vi "CalcShifts.vi"(0 "Sampling Rate (Hz)":dbl=1000000000.0, 1 "c (m/s)":i16=1485, 2 "delay (mm)":sgl, 3 "rf pts":i32, 5 "ROC (m)":dbl=0.012, 7 "# Elements":i16=5, 9 "Radii (m)":sgl[](array[numeric])=[0.0, 0.00132, 0.00142, 0.0019, 0.002, 0.00236, 0.00245, 0.00275, 0.00285, 0.0031], 11 "One Way Receive":bool, 12 "Focal lengths (m)":dbl[](array[numeric])=[0.0085, 0.009, 0.0095, 0.01, 0.0105, 0.011, 0.0115, 0.012, 0.0125, 0.013, 0.0135, 0.014, 0.0145, 0.015], 13 "File index number":i32, 14 "Dual mode":bool) -> (6 "ZoneStart":sgl[](array[numeric]), 8 "ZoneShift":sgl[](array[numeric]), 10 "ZoneLength":sgl[](array[numeric]), 15 "IndexVals":sgl[](array[numeric]))   [LabVIEW 2022 SP3]
panel:
  out "output variable":dbl
  in  "shift":i32
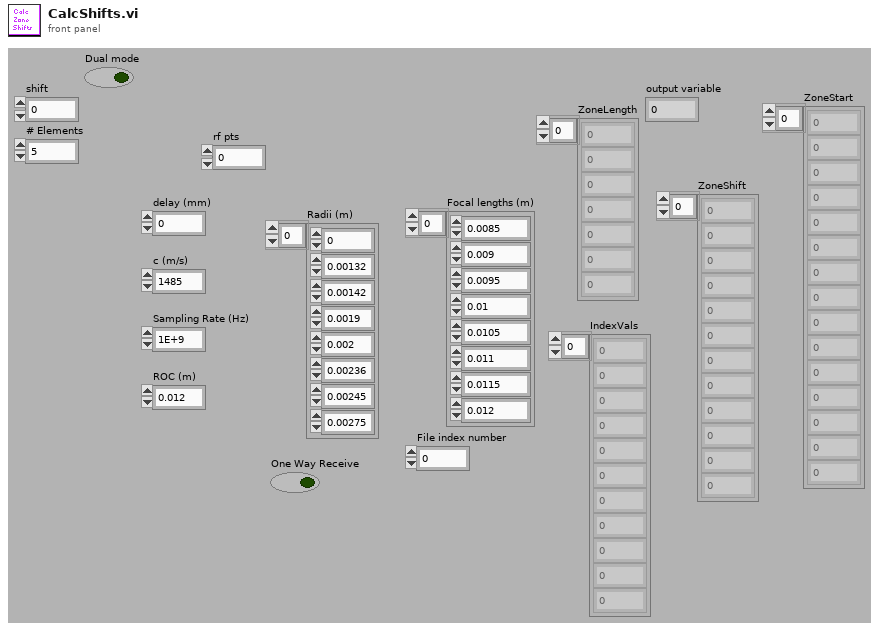
[diagram p1: front panel]
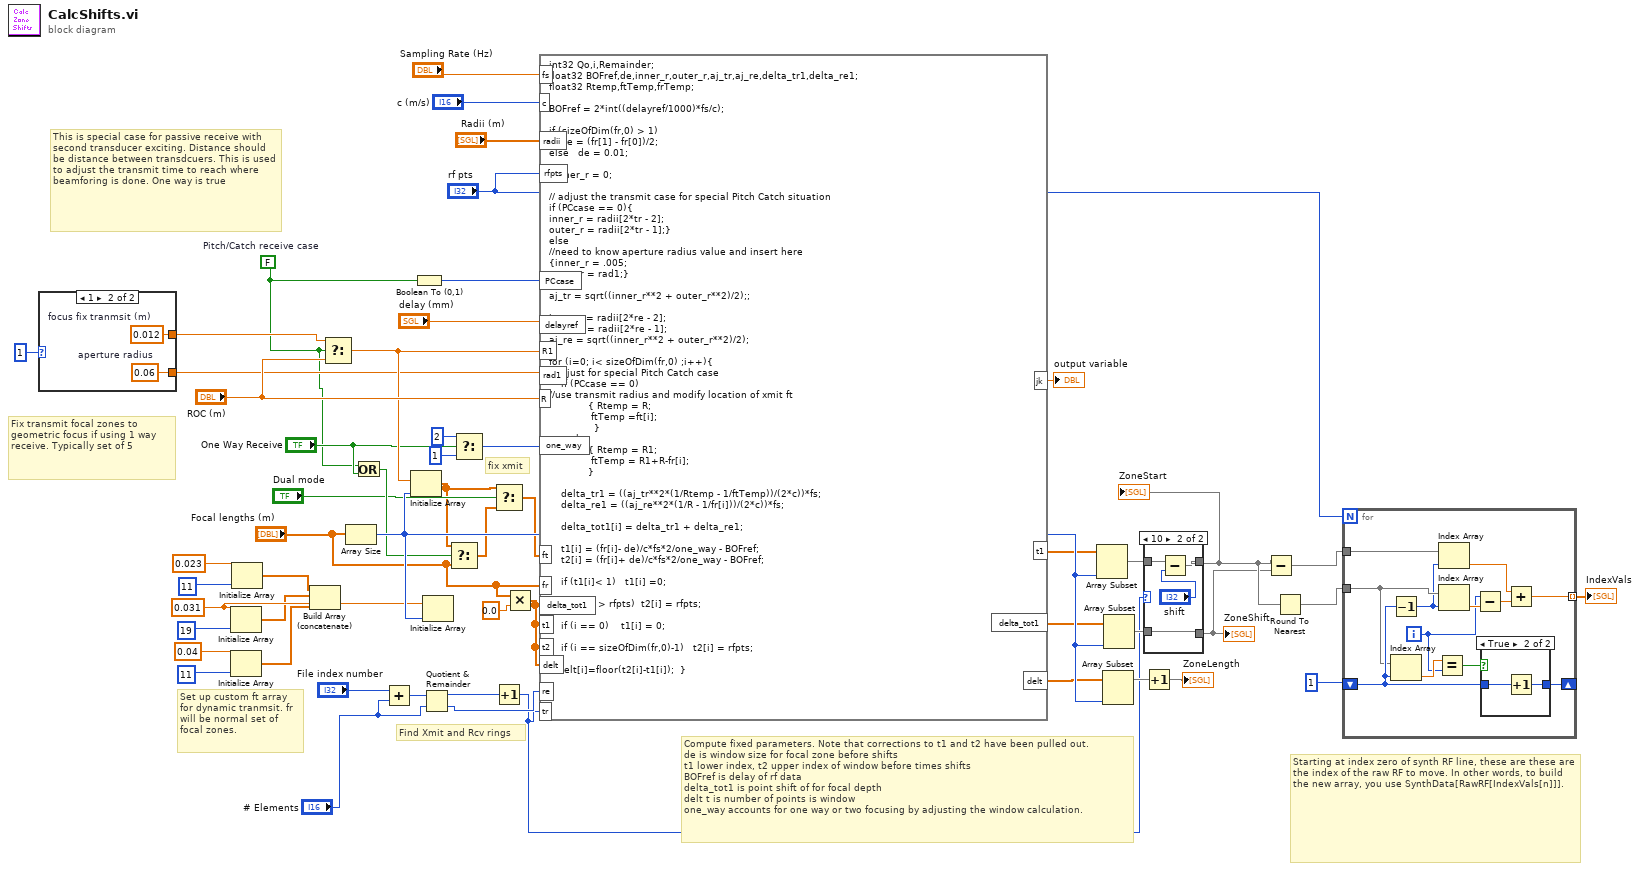
[diagram p0: block diagram]
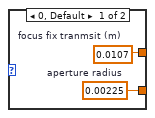
[diagram p2: hidden frame]
diagram:
  w7 = FALSE  # Pitch/Catch receive case
  w50 = 0.031
  # "fix xmit"
  # "This is special case for passive receive with second transducer exciting. Distance should be distance between transdcuers. This is used to adjust the transmit time to reach where beamforing is done. One way is true"
  # "Starting at index zero of synth RF line, these are these are the index of the raw RF to move. In other words, to build the new array, you use SynthData[RawRF[IndexVals[n]]]."
  # "Fix transmit focal zones to geometric focus if using 1 way receive. Typically set of 5"
  # "Set up custom ft array for dynamic tranmsit. fr will be normal set of focal zones."
  # "Find Xmit and Rcv rings"
  # "Compute fixed parameters. Note that corrections to t1 and t2 have been pulled out.\nde is window size for focal zone before shifts\nt1 lower index, t2 upper index of window before times shifts\nBOFref is delay of rf data\ndelta_tot1 is point shift of for focal depth\ndelt t is number of points is window\none_way accounts for one way or two focusing by adjusting the window calculation."
  n1 = case shown="1" 1 {
    tunnel: [w56 w58] -> w14
    tunnel: [w55 w57] -> w12
    frame 0, Default {
      w55 = 0.00225  # aperture radius
      w56 = 0.0107  # focus fix tranmsit (m)
    }
    frame 1 {
      w57 = 0.06  # aperture radius
      w58 = 0.012  # focus fix tranmsit (m)
    }
  }
  n2 = Initialize Array(w50, 19) -> (w48:dbl[])
  n3 = Initialize Array(0.04, 11) -> (w49:dbl[])
  n4 = Initialize Array(0.023, 11) -> (w47:dbl[])
  n5 = Build Array (concatenate)(w47, w48, w49) -> ()  [unwired: 1 out]
  n6 = Select(t=w14, s=w7, f="ROC (m)") -> (s? t:f=w16:dbl)
  n7 = Array Size(array="Focal lengths (m)") -> (size(s)=w52:i32)
  n8 = Or(x=w7, y="One Way Receive") -> (x .or. y?=w9:bool)
  n9 = Add(x="File index number", y="# Elements") -> (x+y=w39:i32)
  n10 = Initialize Array(w16, w52) -> (w1:dbl[])
  n11 = Boolean To (0,1)(Boolean=w7) -> (0, 1=w15:i16)
  n12 = Quotient & Remainder(x=w39, y="# Elements") -> (x-y*floor(x/y)=w40:i32, floor(x/y)=w11:i32)
  n13 = Initialize Array(w50, w52) -> ()  [unwired: 1 out]
  n14 = Select(t=w1, s=w9, f="Focal lengths (m)") -> (s? t:f=w4:dbl[])
  n15 = Select(t=2, s="One Way Receive", f=1) -> (s? t:f=w5:i32)
  n16 = Select(t=w1, s="Dual mode", f=w4) -> (s? t:f=w3:dbl[])
  n17 = Increment(x=w40) -> (x+1=w10:i32)
  n18 = Multiply(x="Focal lengths (m)", y=0.0) -> (x*y=w19:dbl[])
  n19 = formula code="int32 Qo,i,Remainder;\nfloat32 BOFref,de,inner_r,outer_r,aj_tr,aj_re,delta_tr1,delta_re1;\nfloat32 Rtemp,ftTemp,frTemp;\n\nBOFref = 2*int((delayref/1000)*fs/c);\n\nif (sizeOfDim(fr,0) > 1)\n    de = (fr[1] - fr[0])/2;\nelse   de = 0.01;\n\n//inner_r = 0;\n\n// adjust the transmit case for special Pitch Catch situation\nif (PCcase == 0){\ninner_r = radii[2*tr - 2];\nouter_r = radii[2*tr - 1];}\nelse \n//need to know aperture radius value and insert here\n{inner_r = .005;\nouter_r = rad1;}\n\naj_tr = sqrt((inner_r**2 + outer_r**2)/2);;\n\ninner_r = radii[2*re - 2];\nouter_r = radii[2*re - 1];\naj_re = sqrt((inner_r**2 + outer_r**2)/2);\n\nfor (i=0; i< sizeOfDim(fr,0) ;i++){\n//adjust for special Pitch Catch case\n    if (PCcase == 0)\n//use transmit radius and modify location of xmit ft\n             { Rtemp = R;\n              ftTemp =ft[i];\n               }\n       else\n             { Rtemp = R1;\n              ftTemp = R1+R-fr[i];\n             }\n\n    delta_tr1 = ((aj_tr**2*(1/Rtemp - 1/ftTemp))/(2*c))*fs;\n    delta_re1 = ((aj_re**2*(1/R - 1/fr[i]))/(2*c))*fs;\n    \n    delta_tot1[i] = delta_tr1 + delta_re1;\n  \n    t1[i] = (fr[i]- de)/c*fs*2/one_way - BOFref;\n    t2[i] = (fr[i]+ de)/c*fs*2/one_way - BOFref;    \n\n    if (t1[i]< 1)   t1[i] =0;\n   \n    if (t2[i] > rfpts)  t2[i] = rfpts;\n   \n    if (i == 0)    t1[i] = 0;\n\n    if (i == sizeOfDim(fr,0)-1)   t2[i] = rfpts;\n\n   delt[i]=floor(t2[i]-t1[i]);  }"("delayref"="delay (mm)", "radii"="Radii (m)", "fr"="Focal lengths (m)", "fs"="Sampling Rate (Hz)", "rfpts"="rf pts", "tr"=w10, "re"=w11, "c"="c (m/s)", "R"="ROC (m)", "ft"=w3, "one_way"=w5, "delta_tot1"=w19, "t1"=w19, "t2"=w19, "delt"=w19, "R1"=w16, "PCcase"=w15, "rad1"=w12) -> ("t1"=w34:dbl[], "delt"=w36:dbl[], "delta_tot1"=w35:dbl[], "jk"=→"output variable":dbl)
  n20 = Array Subset(array=w34, length=w52) -> (w26:dbl[])  [unwired: 1 in]
  n21 = Array Subset(array=w36, length=w52) -> (w37:dbl[])  [unwired: 1 in]
  n22 = Array Subset(array=w35, length=w52) -> (w24:dbl[])  [unwired: 1 in]
  n23 = case shown="10" w10 {
    tunnel: [w60 w63] -> w25
    tunnel: w26 -> [w60 w64]
    tunnel: [w59 w61] -> w23
    tunnel: w24 -> [w59 w61]
    frame 0, Default {
    }
    frame 10 {
      n24 = Subtract(x=w64, y="shift") -> (x-y=w63:dbl[])
    }
  }
  "ZoneStart" <- w25
  "ZoneShift" <- w23
  n25 = Increment(x=w37) -> (x+1=→"ZoneLength":dbl[])
  n26 = Subtract(x=w25, y=w23) -> (x-y=w29:dbl[])
  n27 = Round To Nearest(number=w25) -> (nearest integer value=w30:dbl[])
  n28 = for {
    N: "rf pts" -> [_]
    tunnel: w29 -> [w76]
    tunnel: w30 -> [w69]
    shift-right: [w73] -> _
    shift-left: 1 -> [w72]
    tunnel: [w70] -> w27 mode=indexing
    i -> [w66]
    n29 = Decrement(x=w72) -> (x-1=w68:i32)
    n30 = Index Array(array=w69, index=w72) -> (element=w75:dbl)
    n31 = Equal?(x=w75, y=w66) -> (x = y?=w74:bool)
    n32 = Index Array(array=w76, index=w68) -> (element=w71:dbl)
    n33 = Index Array(array=w69, index=w68) -> (element=w67:dbl)
    n34 = Subtract(x=w66, y=w67) -> (x-y=w65:dbl)
    n35 = case shown="True" w74 {
      tunnel: w72 -> [w77 w79]
      tunnel: [w77 w78] -> w73
      frame False {
      }
      frame True {
        n36 = Increment(x=w79) -> (x+1=w78:i32)
      }
    }
    n37 = Add(x=w71, y=w65) -> (x+y=w70:dbl)
  }
  "IndexVals" <- w27
